vi "Release.vi"(8 "error in":errorcluster, 11 "File Logger Interface in":refnum<class "CSV Log Type.lvclass">) -> (0 "error out":errorcluster, 3 "File Logger Interface out":refnum<class "CSV Log Type.lvclass">)   [LabVIEW 2020, in "CSV Log Type.lvclass"]
uses:
  CSV Log Type.lvclass
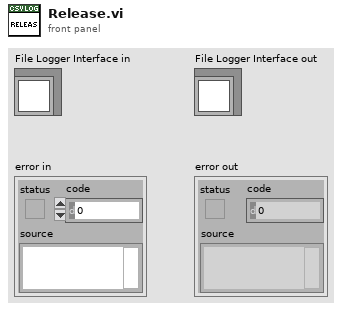
[diagram p1: front panel]
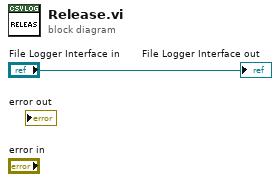
[diagram p0: block diagram]
diagram:
  "File Logger Interface out" <- "File Logger Interface in"
